vi "624 H Drive.vi"(0 "Y Power":dbl, 1 "Center Piston Down?":bool, 5 "Turn Power":dbl, 7 "Strafe Power":dbl, 9 "Y Sensitivity":dbl, 11 "Turn Sensitivity":dbl, 12 "Traction?":bool) -> (4 "HDrive Piston":bool, 6 "Right Motor Output":dbl, 8 "Left Motor Output":dbl, 10 "Center Motor Output":dbl, 15 "Grasshopper Pistons":bool)   [LabVIEW 2016]
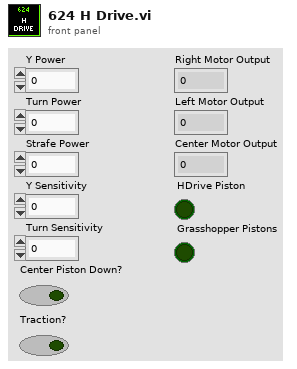
[diagram p1: front panel]
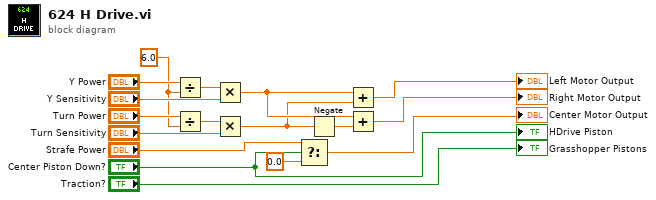
[diagram p0: block diagram]
diagram:
  w11 = 6.0 ("y")
  n1 = Divide(x="Y Power", y=w11) -> (x/y=w16:dbl)
  n2 = Divide(x="Turn Power", y=w11) -> (x/y=w14:dbl)
  n3 = Multiply(x=w16, y="Y Sensitivity") -> (x*y=w10:dbl)
  n4 = Multiply(x=w14, y="Turn Sensitivity") -> (x*y=w9:dbl)
  n5 = Select(t="Strafe Power", s="Center Piston Down?", f=0.0) -> (s? t:f=→"Center Motor Output":dbl)
  n6 = Negate(x=w9) -> (-x=w6:dbl)
  n7 = Add(x=w10, y=w9) -> (x+y=→"Left Motor Output":dbl)
  n8 = Add(x=w10, y=w6) -> (x+y=→"Right Motor Output":dbl)
  "HDrive Piston" <- "Center Piston Down?"
  "Grasshopper Pistons" <- "Traction?"
